vi "Destroy.vi"(8 "error in (no error)":errorcluster, 11 "logger in":refnum<class "Logger.lvclass">) -> (0 "error out":errorcluster, 3 "failure info":T1 {"Log Record"."timestamp" format="%<%x %.3X>T"})   [LabVIEW 2018, in "GLog.lvlib" / "Logger.lvclass"]
uses:
  Logger.lvclass
  Failure Information.ctl
  Log Record.ctl
  Internal Log Levels.ctl
  Logger.lvclass/Logger.ctl
  extension/formatting_handler_interface/Formatting Handler.lvclass
  GLog.lvlib
panel:
  # "Connector Pane"
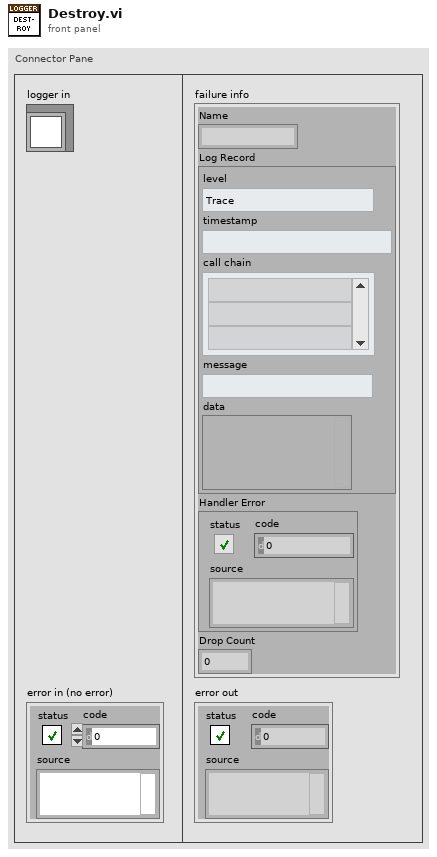
[diagram p1: front panel]
types:
  T1 = typedef "GLog.lvlib/Failure Information.ctl" = cluster{"Name":string, "Log Record":T2, "Handler Error":errorcluster, "Drop Count":u32}
  T2 = typedef "GLog.lvlib/Log Record.ctl" = cluster{"level":T3, "timestamp":timestamp, "call chain":string[], "message":string, "data":variant}
  T3 = typedef "GLog.lvlib/Internal Log Levels.ctl" = enum16{"Trace", "Debug", "Info", "Warning", "Error", "Critical", "Internal"}
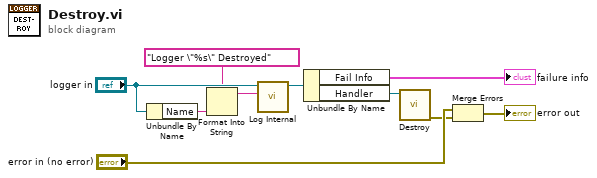
[diagram p0: block diagram]
diagram:
  n1 = Unbundle By Name("logger in") -> ("Name"=w1:string)
  n2 = Format Into String(format string="Logger \"%s\" Destroyed" ("message"), w1) -> (resulting string=w2:string)  [unwired: 2 in, 1 out]
  n3 = call "Log Internal.vi"("message"=w2, "logger in"="logger in") -> ("logger out"=w7:refnum<class "Logger.lvclass">)  [unwired: 9 in]
  n4 = Unbundle By Name(w7) -> ("Fail Info"=→"failure info":T1, "Handler"=w10:refnum<class "Formatting Handler.lvclass">)
  n5 = call-dynamic "Destroy.vi"("handler in"=w10) -> ("error out"=w8:errorcluster)  [unwired: 10 in]
  n6 = Merge Errors("error in (no error)", w8) -> (→"error out":errorcluster)
